vi "Wheel Sensor.vi"(4 "Reset":bool, 8 "0 Outside Loop":dbl, 11 "Input":bool) -> (0 "0 Shift Register Loop":dbl)   [LabVIEW 2015]
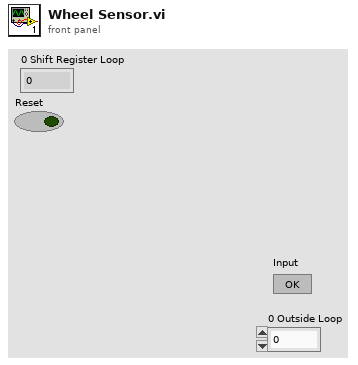
[diagram p1: front panel]
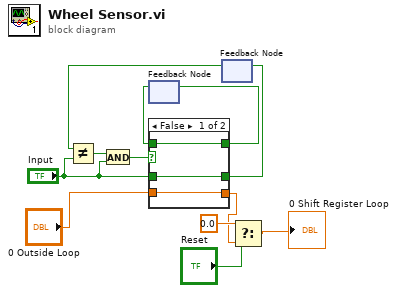
[diagram p0: block diagram]
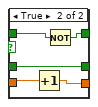
[diagram p2: hidden frame]
diagram:
  n1 = feedback #1() -> (w12:bool)  [unwired: 1 in]
  n2 = feedback #2() -> (w9:bool)  [unwired: 1 in]
  n3 = Not Equal?(x=w9, y="Input") -> (x != y?=w8:bool)
  n4 = And(x=w8, y="Input") -> (x .and. y?=w7:bool)
  n5 = case shown="False" w7 {
    tunnel: w12 -> [w15 w20]
    tunnel: [w15 w19] -> w11
    tunnel: [w14 w18] -> w10
    tunnel: "Input" -> [w14 w18]
    tunnel: "0 Outside Loop" -> [w13 w17]
    tunnel: [w13 w16] -> w2
    frame False {
    }
    frame True {
      n6 = Increment(x=w17) -> (x+1=w16:dbl)
      n7 = Not(x=w20) -> (.not. x?=w19:bool)
    }
  }
  n8 = feedback-in #1(w11) -> ()
  n9 = feedback-in #2(w10) -> ()
  n10 = Select(t=0.0, s="Reset", f=w2) -> (s? t:f=→"0 Shift Register Loop":dbl)
